vi "Add When VIs.vi"(8 "error in (no error)":errorcluster, 11 "Mock Class Generator In":refnum<class "Pure Mock Class Generator.lvclass">) -> (0 "error out":errorcluster, 2 "When VIs":path[](array[path]), 3 "Mock Class Generator Out":refnum<class "Pure Mock Class Generator.lvclass">)   [LabVIEW 2020]
uses:
  Pure Mock Class Generator.lvclass
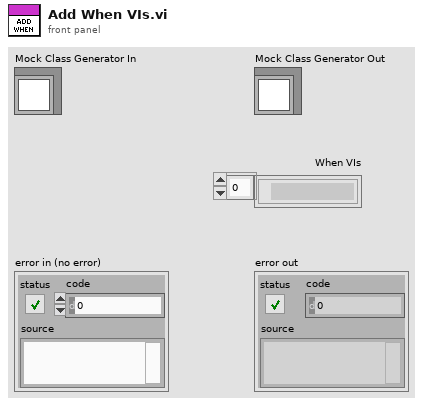
[diagram p1: front panel]
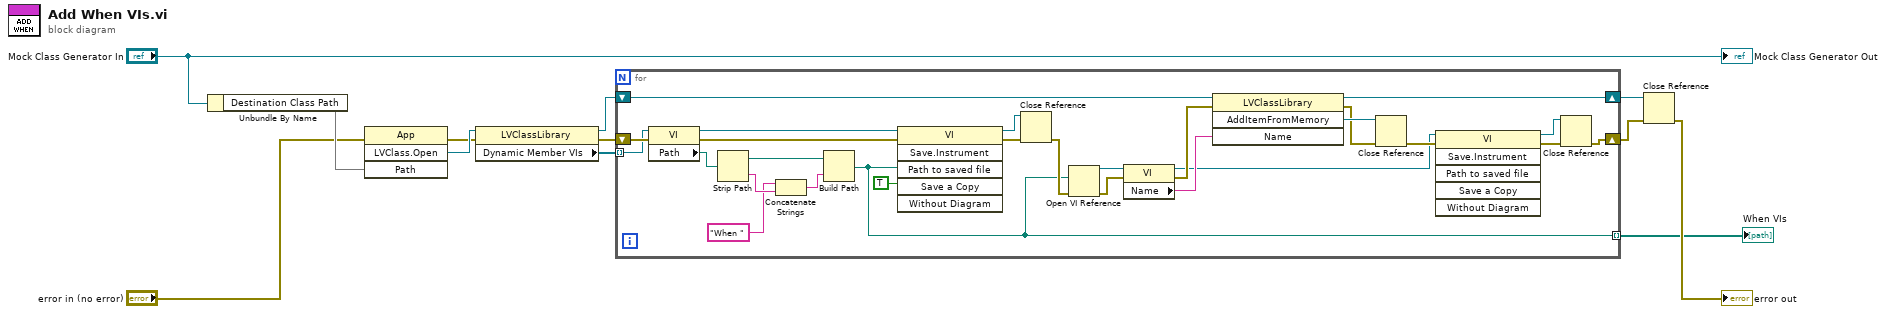
[diagram p0: block diagram]
diagram:
  n1 = Unbundle By Name("Mock Class Generator In") -> ("Destination Class Path"=w8)
  n2 = invoke class="App" method="LVClass.Open"(error in="error in (no error)", "Path"=w8) -> (error out=w11:errorcluster, "LVClass.Open"=w12:refnum<vi>)  [unwired: 2 in, 2 out]
  n3 = property class="LVClassLibrary"(reference=w12, error in=w11) -> (reference out=w6:refnum<vi>, error out=w10:errorcluster, "Dynamic Member VIs"=w7:refnum<vi>[])
  n4 = for {
    tunnel: w7 -> [w32] mode=indexing
    shift-right: [w14] -> w4
    shift-left: w10 -> [w33]
    shift-right: [w21] -> w5
    shift-left: w6 -> [w25]
    tunnel: [w13] -> w1 mode=indexing
    n5 = property class="VI"(reference=w32, error in=w33) -> (reference out=w37:refnum<vi>, error out=w36:errorcluster, "Path"=w39:path)
    n6 = Strip Path(path=w39) -> (stripped path=w31:path, name=w30:string)
    n7 = Concatenate Strings("When " ("string"), w30) -> (w28:string)
    n8 = Build Path(base path=w31, name or relative path=w28) -> (appended path=w13:path)
    n9 = invoke class="VI" method="Save.Instrument"(reference=w37, error in=w36, "Path to saved file"=w13, "Save a Copy"=TRUE) -> (reference out=w34:refnum<vi>, error out=w35:errorcluster)  [unwired: 2 in, 4 out]
    n10 = Close Reference(reference=w34, error in (no error)=w35) -> (error out=w24:errorcluster)
    n11 = Open VI Reference(vi path=w13, error in (no error)=w24) -> (vi reference=w23:refnum<vi>, error out=w22:errorcluster)  [unwired: 4 in]
    n12 = property class="VI"(reference=w23, error in=w22) -> (reference out=w15:refnum<vi>, error out=w26:errorcluster, "Name"=w27:string)
    n13 = invoke class="LVClassLibrary" method="AddItemFromMemory"(reference=w25, error in=w26, "Name"=w27) -> (reference out=w21:refnum<vi>, error out=w17:errorcluster, "AddItemFromMemory"=w18:refnum<vi>)  [unwired: 1 in, 1 out]
    n14 = Close Reference(reference=w18, error in (no error)=w17) -> (error out=w16:errorcluster)
    n15 = invoke class="VI" method="Save.Instrument"(reference=w15, error in=w16) -> (reference out=w20:refnum<vi>, error out=w19:errorcluster)  [unwired: 4 in, 4 out]
    n16 = Close Reference(reference=w20, error in (no error)=w19) -> (error out=w14:errorcluster)
  }
  "When VIs" <- w1
  n17 = Close Reference(reference=w5, error in (no error)=w4) -> (error out=→"error out":errorcluster)
  "Mock Class Generator Out" <- "Mock Class Generator In"
